vi "BlueSimpleReachTask - Front panel timer.vi"() -> ()   [LabVIEW 2010]
uses:
  Controls/Bits to Write.ctl
panel:
  in  "Use Arm Freeze Counter":bool
  out "Arm Freeze Counter":dbl
  in  "Catch probability":i32 min=0 max=100 step=1
  out "Catch Trial?":bool
  in  "Catch Trial":bool
  out "DO Task":refnum<k21>="BlueSimple_DO_All"
  out "DI Task":refnum<k21>="BlueSimple_DI"
  out "Exp correct":i32
  out "Record flag":bool
  in  "Recenter motor":bool
  in  "Override bumps":bool
  in  "Start bump timer?":bool
  in  "Trial type":u16(ring) items=["Allflash/sensory", "Precue/memory"]
  in  "DBS On?":bool
  in  "Home+target OK?":bool
  out "Exp reset":bool
  out "target set #":i32
  in  "duration (s)":dbl=0.18 format="%.4f"
  in  "Inter-pulse delay":cluster{"Fix":dbl, "Rnd":dbl}={"Fix"=0.0, "Rnd"=1.5} {"Rnd" format="%.4f"; "Fix" format="%_4g"}
  in  "Autofeed?":bool
  out "Just initialized\nhold loop?":bool
  in  "Home reward?":bool
  in  "Home reward":cluster{"Fix":dbl, "Rnd":dbl} {"Rnd" format="%.4f"; "Fix" format="%_4g"}
  in  "Override 4":bool caption="Override 1"
  in  "Override 3":bool caption="Override 1"
  in  "Override 2":bool=TRUE caption="Override 1"
  in  "Override 1":bool=TRUE
  in  "LED lines":T1={"LED1"=1, "LED2"=2, "LED3"=3, "LED4"=4}
  in  "LED1":i16=5
  in  "LED2":i16=6
  in  "LED3":i16=7
  in  "LED4":i16=8
  in  "Bump Parameters":T2={"Distance (deg)"=2.0, "Travel time (ms)"=500.0} {"Travel time (ms)" min=0.1 max=10000.0; "Distance (deg)" min=0.1}
  in  "Bump delay":cluster{"Fix":dbl, "Rnd":dbl}={"Fix"=2.0, "Rnd"=8.0} {"Rnd" format="%.4f"; "Fix" format="%_4g"}
  in  "Sine parameters":T3={"Frequency"=1.0, "Degrees\npk-pk"=8.0, "Cycles"=10000} {"Degrees\npk-pk" min=0.1 max=120.0; "Frequency" min=0.001 format="%#_4g"}
  in  "Home":bool
  in  "Bumps":bool
  in  "Sines?":bool
  out "target set size":i32
  out "# target sets":u16
  in  "# Cycles":i16=20
  out "Instruct duration":dbl format="%.4f"
  out "Pre-I hold":dbl format="%.4f"
  out "Touching target\nlast time?":bool
  in  "Rand/Seq?":bool=TRUE
  in  "Target set":i16[](array[ring]) items=["1", "2", "3", "4"]
  in  "Block":T4(array[cluster])=array[6501 elements]
  in  "Settings In":T5={"Pre-I hold"={"Fixed (s)"=0.5, "Random (s)"=0.5}, "LED I duration"={"Fixed (s)"=0.5, "Random (s)"=0.0}, "All Flash?"=FALSE, "Pre-cue brightness"=0, "Post-I hold"={"Fixed (s)"=0.7, "Random (s)"=0.3}, "Post-I \nbounce-off"={"Fixed (s)"=0.3, "Random (s)"=0.0}, "Capture timeout"={"Fixed (s)"=1.5, "Random (s)"=0.0}, "Tone duration"={"Fixed (s)"=0.5, "Random (s)"=0.0}, "LED C duration"={"Fixed (s)"=0.5, "Random (s)"=0.0}, "Cue brightness"=0, "Hold duration"={"Fixed (s)"=0.3, "Random (s)"=0.0}, "Allowed\nbounce-off"={"Fixed (s)"=0.2, "Random (s)"=0.0}, "Post-capture brightness"=0, "Reward duration"={"Fixed (s)"=0.7, "Random (s)"=0.0}, "Intertrial interval"={"Fixed (s)"=0.5, "Random (s)"=0.0}, "Persistent Mode?"=FALSE, "Error bong?"=TRUE, "Critter"=0, "Blocks"=[], "Target set"=[], "Rand/Seq?"=TRUE, "Trial type"=0, "Sines?"=FALSE, "Bumps"=FALSE, "Sine parameters"={"Frequency"=0.25, "Degrees\npk-pk"=6.0, "Cycles"=10000}, "Bump timing"={"Fix"=2.0, "Rnd"=8.0}, "Bump Parameters"={"Distance (deg)"=2.0, "Travel time (ms)"=500.0}, "DBS On?"=FALSE, "Home reward?"=FALSE, "Home+target OK?"=FALSE} {"Bump Parameters"."Travel time (ms)" min=0.1 max=10000.0; "Bump Parameters"."Distance (deg)" min=0.1; "Bump timing"."Rnd" format="%.4f"; "Bump timing"."Fix" format="%_4g"; "Sine parameters"."Degrees\npk-pk" min=0.1 max=120.0; "Sine parameters"."Frequency" min=0.001 format="%#_4g"; "Trial type" items=["Allflash/sensory", "Precue/memory"]; "Target set" items=["1", "2", "3", "4"]; "Critter" items=["Mojo", "Smokey"]; "Post-I \nbounce-off"."Random (s)" format="%.4f"; "Post-I \nbounce-off"."Fixed (s)" format="%_4g"; "Allowed\nbounce-off"."Random (s)" format="%.4f"; "Allowed\nbounce-off"."Fixed (s)" format="%_4g"; "LED C duration"."Random (s)" format="%.4f"; "LED C duration"."Fixed (s)" format="%.4f"; "Capture timeout"."Random (s)" format="%.4f"; "Capture timeout"."Fixed (s)" format="%.4f"; "Post-I hold"."Random (s)" format="%.4f"; "Post-I hold"."Fixed (s)" format="%.4f"; "Hold duration"."Random (s)" format="%.4f"; "Hold duration"."Fixed (s)" format="%_4g"; "Intertrial interval"."Random (s)" format="%.4f"; "Intertrial interval"."Fixed (s)" format="%.4f"; "Reward duration"."Random (s)" format="%.4f"; "Reward duration"."Fixed (s)" format="%.4f"; "LED I duration"."Random (s)" format="%.4f"; "LED I duration"."Fixed (s)" format="%.4f"; "Tone duration"."Random (s)" format="%.4f"; "Tone duration"."Fixed (s)" format="%.4f"; "Pre-I hold"."Random (s)" format="%.4f"; "Pre-I hold"."Fixed (s)" format="%_4g"}
  in  "pause":bool
  out "Assign settings":bool
  out "current path":path
  out "next trial path":path
  in  "Critter":u16(ring) items=["Mojo", "Smokey", "Blue", "Odo", "Monk 5", "Monk 6", "Monk 7", "Monk 8", "Monk 9", "Monk 10"]
  out "Total incorrect":i32
  in  "Write Settings":bool
  in  "Read Settings":bool
  in  "All Flash?":bool
  in  "Post-capture brightness":i16 caption="Brightness"
  in  "Cue brightness":i16=6 caption="Brightness"
  in  "Pre-cue brightness":i16 caption="Brightness"
  out "Total correct":i32
  out "Total %":dbl
  out "Total trials":i32
  in  "Error\nbong?":bool=TRUE
  out "TS Home":bool
  out "TS 4":bool
  out "TS 3":bool
  out "TS 2":bool
  out "TS 1":bool
  out "Waveform Chart":T6(graph)
  out "Block trials":i32
  out "Block %":dbl
  in  "Reset\ncounters":bool
  in  "Post-I \nbounce-off":cluster{"Fix":dbl, "Rnd":dbl}={"Fix"=0.3, "Rnd"=0.0} caption="Allowed\nbounce-off" {"Rnd" format="%.4f"; "Fix" format="%_4g"}
  out "Exp trials":i32
  out "Exp %":dbl
  in  "Touch lines":T7={"Home touch"=0, "Touch 1"=1, "Touch 2"=2, "Touch 3"=3, "Touch 4"=4}
  out "Current stage":T8(ring)
  in  "Allowed\nbounce-off":cluster{"Fix":dbl, "Rnd":dbl}={"Fix"=0.2, "Rnd"=0.0} {"Rnd" format="%.4f"; "Fix" format="%_4g"}
  in  "LED C duration":cluster{"Fix":dbl, "Rnd":dbl}={"Fix"=0.5, "Rnd"=0.0} caption="LED duration" {"Rnd" format="%.4f"; "Fix" format="%.4f"}
  in  "Capture timeout":cluster{"Fix":dbl, "Rnd":dbl}={"Fix"=1.5, "Rnd"=0.0} caption="Response time" {"Rnd" format="%.4f"; "Fix" format="%.4f"}
  in  "Post-I hold":cluster{"Fix":dbl, "Rnd":dbl}={"Fix"=0.5, "Rnd"=0.5} {"Rnd" format="%.4f"; "Fix" format="%.4f"}
  out "Last trial successful?":bool
  in  "Persistent\n Mode?":bool
  in  "Touch 4":i16=4
  in  "Touch 3":i16=3
  in  "Touch 2":i16=2
  in  "Touch 1":i16=1
  in  "Home touch":i16
  in  "Hold duration":cluster{"Fix":dbl, "Rnd":dbl}={"Fix"=0.3, "Rnd"=0.0} {"Rnd" format="%.4f"; "Fix" format="%_4g"}
  out "Target":i16
  in  "stop":bool
  in  "device":i16=1
  in  "line direction map":i32=2147483616 format="%.0b"
  out "DIGIO task ID":u32 format="%.0x"
  out "error out":errorcluster
  in  "Intertrial interval":cluster{"Fix":dbl, "Rnd":dbl}={"Fix"=0.5, "Rnd"=0.0} {"Rnd" format="%.4f"; "Fix" format="%.4f"}
  in  "Reward duration":cluster{"Fix":dbl, "Rnd":dbl}={"Fix"=0.7, "Rnd"=0.0} {"Rnd" format="%.4f"; "Fix" format="%.4f"}
  in  "LED I duration":cluster{"Fix":dbl, "Rnd":dbl}={"Fix"=0.5, "Rnd"=0.0} caption="LED duration" {"Rnd" format="%.4f"; "Fix" format="%.4f"}
  in  "Tone duration":cluster{"Fix":dbl, "Rnd":dbl}={"Fix"=0.5, "Rnd"=0.0} {"Rnd" format="%.4f"; "Fix" format="%.4f"}
  in  "Pre-I hold":cluster{"Fix":dbl, "Rnd":dbl}={"Fix"=0.5, "Rnd"=0.5} {"Rnd" format="%.4f"; "Fix" format="%_4g"}
  # "Auto-feed"
  # "DBS"
  # "Pre-\ninstruction\nhold"
  # "Post-\ninstruction\nhold"
  # "Instruction"
  # "Target capture"
  # "Target hold"
  # "Reward"
  # "Intertrial"
  # "Motor"
  # "Override"
  # "+"
  # "+"
  # "+"
  # "Pre-\ninstruction\nhold"
  # "Instruction"
  # "Post-\ninstruction\nhold"
  # "Target capture"
  # "Target hold"
  # "Reward"
  # "Intertrial"
  # "+"
  # "+"
  # "+"
  # "+"
  # "+"
  # "+"
  # "+"
  # "+"
  # "+"
  # "+"
  # "+"
  # "+"
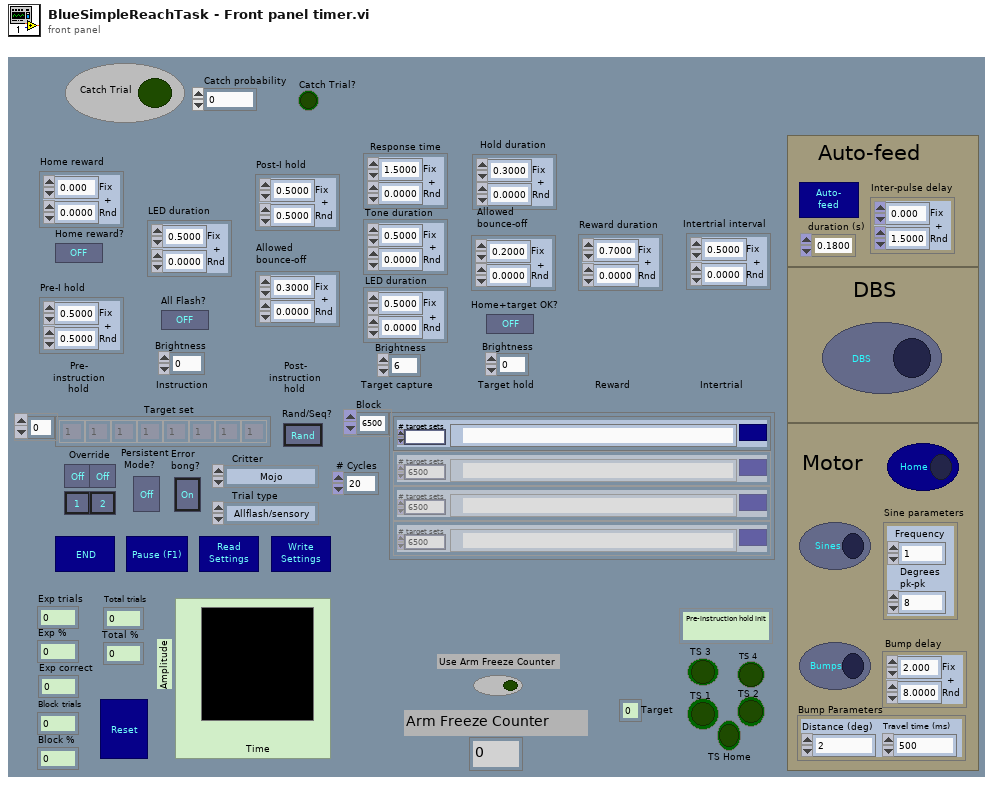
[diagram p1: front panel]
types:
  T1 = cluster{"LED1":i16, "LED2":i16, "LED3":i16, "LED4":i16}
  T2 = cluster{"Distance (deg)":dbl, "Travel time (ms)":dbl}
  T3 = cluster{"Frequency":dbl, "Degrees\npk-pk":dbl, "Cycles":i16}
  T4 = cluster{"Settings file":path, "# target sets":u16}[]
  T5 = cluster{"Pre-I hold":cluster{"Fixed (s)":dbl, "Random (s)":dbl}, "LED I duration":cluster{"Fixed (s)":dbl, "Random (s)":dbl}, "All Flash?":bool, "Pre-cue brightness":i16, "Post-I hold":cluster{"Fixed (s)":dbl, "Random (s)":dbl}, "Post-I \nbounce-off":cluster{"Fixed (s)":dbl, "Random (s)":dbl}, "Capture timeout":cluster{"Fixed (s)":dbl, "Random (s)":dbl}, "Tone duration":cluster{"Fixed (s)":dbl, "Random (s)":dbl}, "LED C duration":cluster{"Fixed (s)":dbl, "Random (s)":dbl}, "Cue brightness":i16, "Hold duration":cluster{"Fixed (s)":dbl, "Random (s)":dbl}, "Allowed\nbounce-off":cluster{"Fixed (s)":dbl, "Random (s)":dbl}, "Post-capture brightness":i16, "Reward duration":cluster{"Fixed (s)":dbl, "Random (s)":dbl}, "Intertrial interval":cluster{"Fixed (s)":dbl, "Random (s)":dbl}, "Persistent Mode?":bool, "Error bong?":bool, "Critter":u16, "Blocks":cluster{"Settings file":path, "# target sets":dbl}[], "Target set":i16[], "Rand/Seq?":bool, "Trial type":u16, "Sines?":bool, "Bumps":bool, "Sine parameters":cluster{"Frequency":dbl, "Degrees\npk-pk":dbl, "Cycles":i16}, "Bump timing":cluster{"Fix":dbl, "Rnd":dbl}, "Bump Parameters":cluster{"Distance (deg)":dbl, "Travel time (ms)":dbl}, "DBS On?":bool, "Home reward?":bool, "Home+target OK?":bool}
  T6 = cluster{"Segment Percentage":dbl, "Total % correct":dbl}
  T7 = cluster{"Home touch":i16, "Touch 1":i16, "Touch 2":i16, "Touch 3":i16, "Touch 4":i16}
  T8 = enum16{"Pre-instruction hold init", "Pre-instruction hold", "Instruction init", "Instruction", "Post-instruction hold init", "Post-instruction hold", "Target capture init", "Target capture", "Target hold init", "Target hold", "Reward stage", "Intertrial"}
  T9 = typedef "Bits to Write.ctl" = enum16{"LED 1 on", "LED 1 off", "LED 2 on", "LED 2 off", "LED 3 on", "LED 3 off", "LED 4 on", "LED 4 off", "All LEDs on", "All LEDs off", "In trial on", "In trial off", "Buzzer on", "Buzzer off", "Reward on", "Reward off", "Target number", "Trial type preQ on", "Trial type preQ off", "Error on", "Error off", "Trial number", "DBS on", "DBS off", "Sine on", "Sine off", "All Bits On", "All Bits Off", "Init", "Specify mask/pattern"}
  T10 = enum16{"Reset", "Increment", "Reset for exp", "Initialize"}
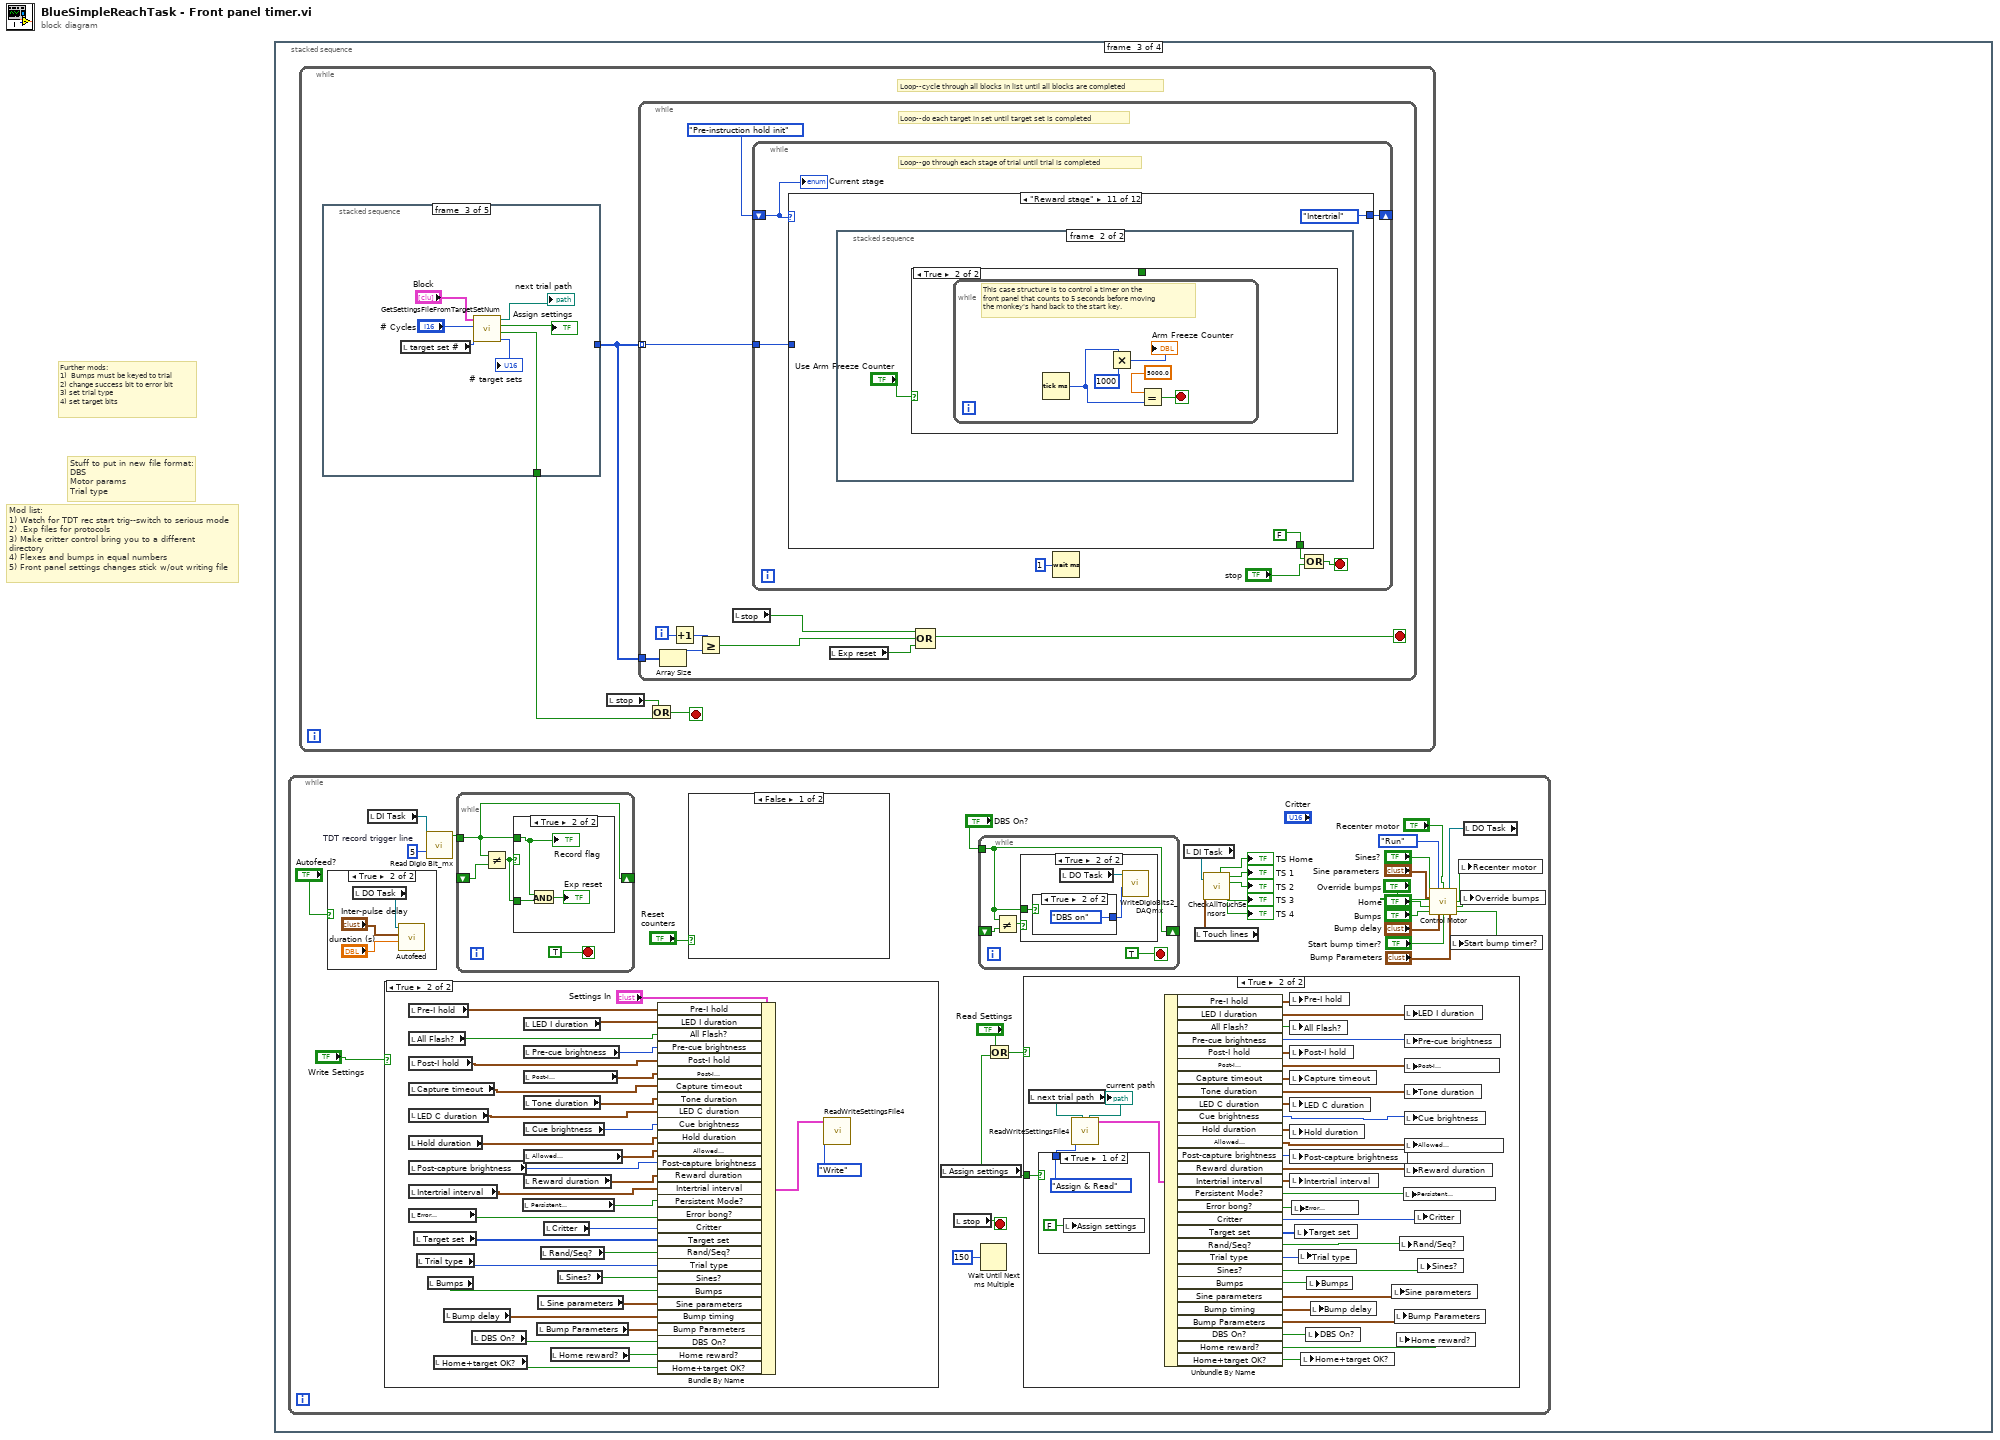
[diagram p0: block diagram]
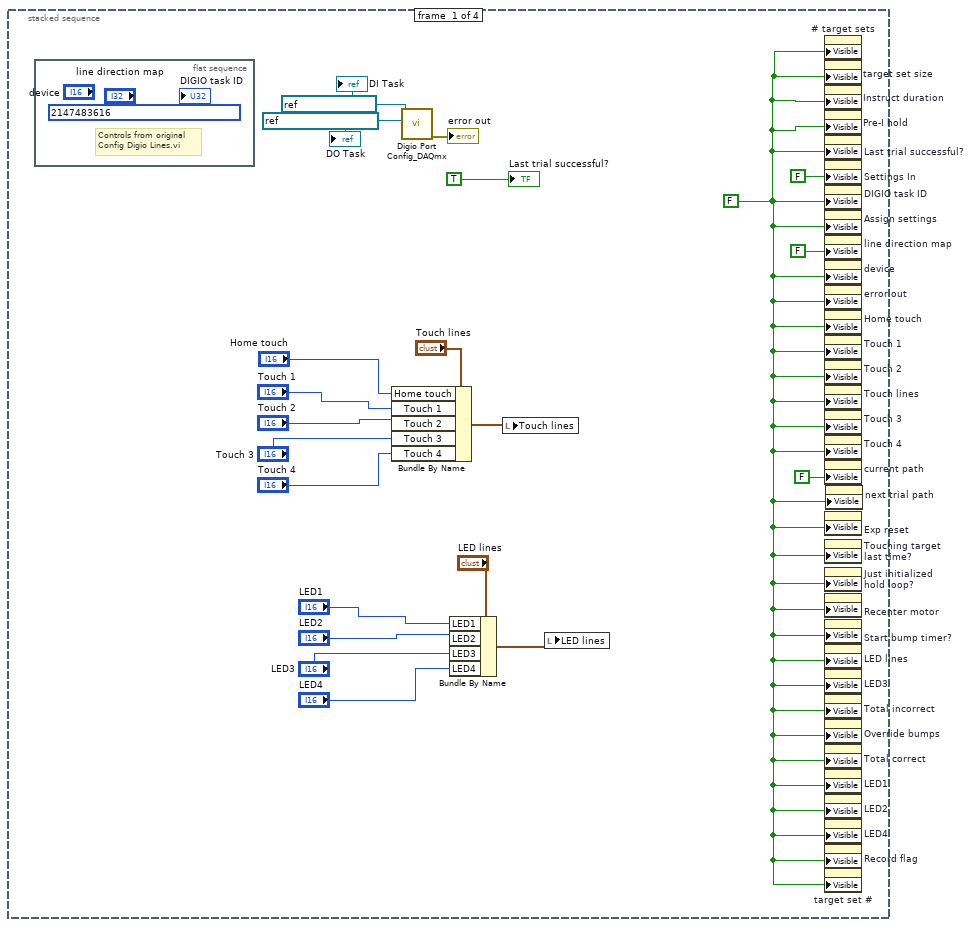
[diagram p2: hidden frame]
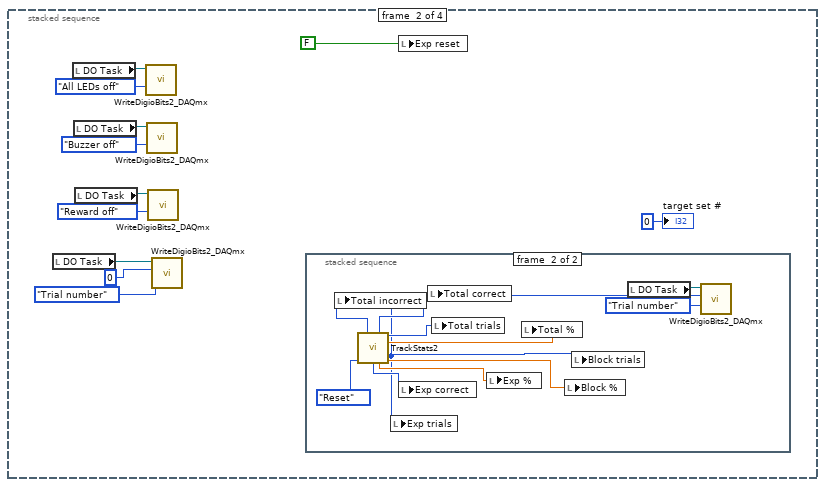
[diagram p3: hidden frame]
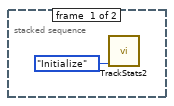
[diagram p4: hidden frame]
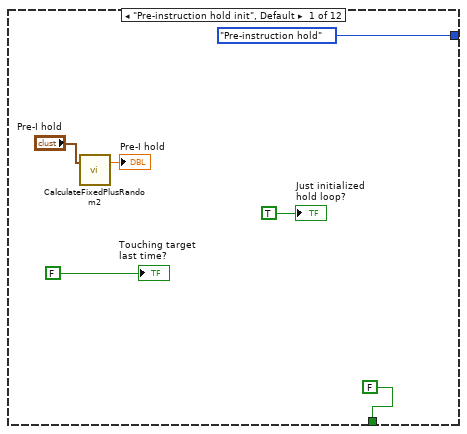
[diagram p5: hidden frame]
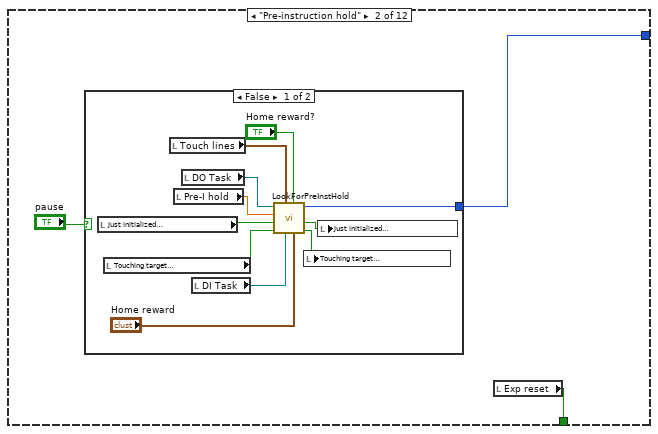
[diagram p6: hidden frame]
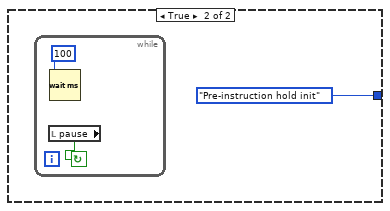
[diagram p7: hidden frame]
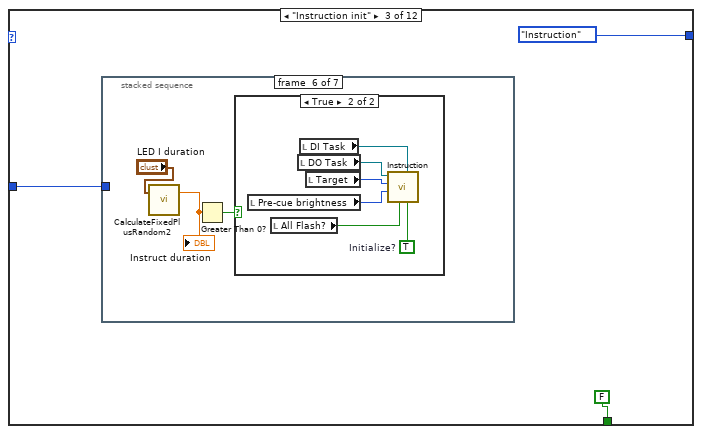
[diagram p8: hidden frame]
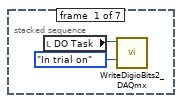
[diagram p9: hidden frame]
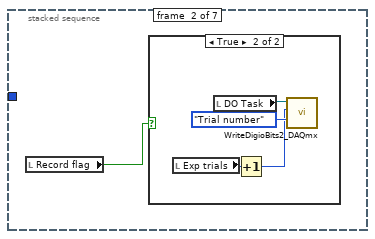
[diagram p10: hidden frame]
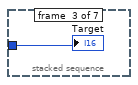
[diagram p12: hidden frame]
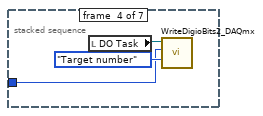
[diagram p13: hidden frame]
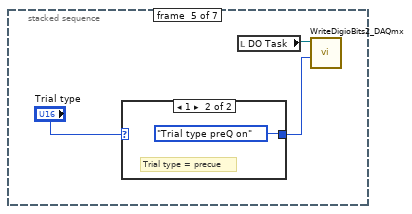
[diagram p14: hidden frame]
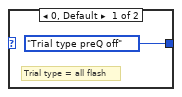
[diagram p15: hidden frame]
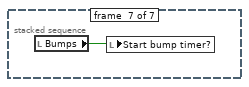
[diagram p17: hidden frame]
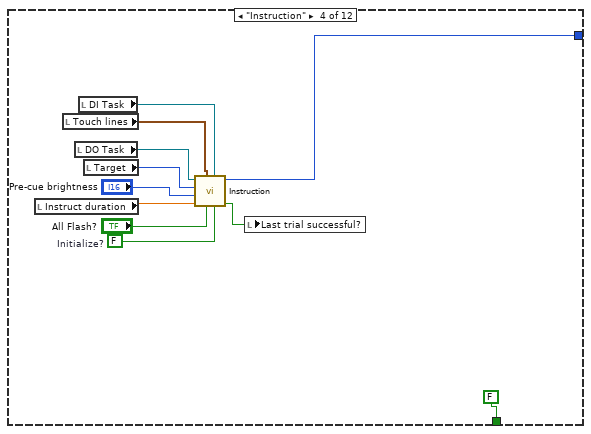
[diagram p18: hidden frame]
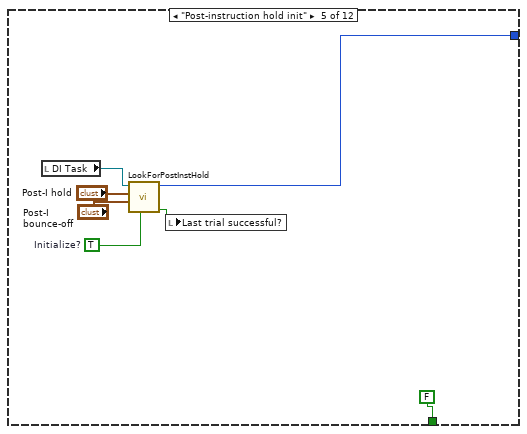
[diagram p19: hidden frame]
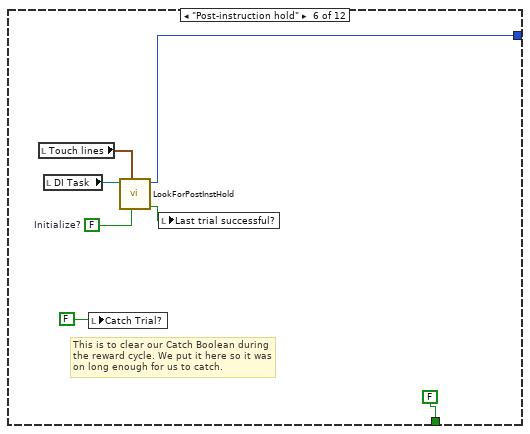
[diagram p20: hidden frame]
diagram:
  # "Stuff to put in new file format:\nDBS\nMotor params\nTrial type"
  # "Further mods:\n1)  Bumps must be keyed to trial\n2) change success bit to error bit\n3) set trial type\n4) set target bits"
  # "Mod list:\n1) Watch for TDT rec start trig--switch to serious mode\n2) .Exp files for protocols\n3) Make critter control bring you to a different directory\n4) Flexes and bumps in equal numbers\n5) Front panel settings changes stick w/out writing file"
  n1 = stacked-sequence {
    frame #0 {
      w2 = refnum<k21> "BlueSimple_DO_All" ("DO Task")
      w3 = refnum<k21> "BlueSimple_DI" ("DI Task")
      w4 = FALSE ("Persistent Mode?")
      n2 = flat-sequence {
        frame #0 {
          (unwired) 2147483616 ("line direction map")
          # "Controls from original\nConfig Digio Lines.vi"
        }
      }
      n3 = Bundle By Name(cluster="Touch lines", "Home touch"="Home touch", "Touch 1"="Touch 1", "Touch 2"="Touch 2", "Touch 3"="Touch 3", "Touch 4"="Touch 4") -> (w20:T7)
      n4 = call "Digio Port Config_DAQmx.vi"("DO Task"=w2, "DI Task"=w3) -> ("error out"=→"error out":errorcluster)  [unwired: 7 in]
      n5 = Bundle By Name(cluster="LED lines", "LED1"="LED1", "LED2"="LED2", "LED3"="LED3", "LED4"="LED4") -> (w8:T1)
      n6 = local write "Touch lines"(w20) -> ()
      n7 = local write "LED lines"(w8) -> ()
      n8 = property on="# target sets" class="DigNum (strict)"("Visible"=w4) -> ()  [unwired: 2 in, 2 out]
      n9 = property on="target set size" class="DigNum (strict)"("Visible"=w4) -> ()  [unwired: 2 in, 2 out]
      n10 = property on="Instruct duration" class="DigNum (strict)"("Visible"=w4) -> ()  [unwired: 2 in, 2 out]
      n11 = property on="Pre-I hold" class="DigNum (strict)"("Visible"=w4) -> ()  [unwired: 2 in, 2 out]
      n12 = property on="Last trial successful?" class="Bool (strict)"("Visible"=w4) -> ()  [unwired: 2 in, 2 out]
      n13 = property on="Settings In" class="Clust (strict)"("Visible"=FALSE) -> ()  [unwired: 2 in, 2 out]
      n14 = property on="DIGIO task ID" class="DigNum (strict)"("Visible"=w4) -> ()  [unwired: 2 in, 2 out]
      n15 = property on="Assign settings" class="Bool (strict)"("Visible"=w4) -> ()  [unwired: 2 in, 2 out]
      n16 = property on="line direction map" class="DigNum (strict)"("Visible"=FALSE) -> ()  [unwired: 2 in, 2 out]
      n17 = property on="device" class="DigNum (strict)"("Visible"=w4) -> ()  [unwired: 2 in, 2 out]
      n18 = property on="error out" class="Clust (strict)"("Visible"=w4) -> ()  [unwired: 2 in, 2 out]
      n19 = property on="Home touch" class="DigNum (strict)"("Visible"=w4) -> ()  [unwired: 2 in, 2 out]
      n20 = property on="Touch 1" class="DigNum (strict)"("Visible"=w4) -> ()  [unwired: 2 in, 2 out]
      n21 = property on="Touch 2" class="DigNum (strict)"("Visible"=w4) -> ()  [unwired: 2 in, 2 out]
      n22 = property on="Touch lines" class="Clust (strict)"("Visible"=w4) -> ()  [unwired: 2 in, 2 out]
      n23 = property on="Touch 3" class="DigNum (strict)"("Visible"=w4) -> ()  [unwired: 2 in, 2 out]
      n24 = property on="Touch 4" class="DigNum (strict)"("Visible"=w4) -> ()  [unwired: 2 in, 2 out]
      n25 = property on="current path" class="Path"("Visible"=FALSE) -> ()  [unwired: 2 in, 2 out]
      n26 = property on="Exp reset" class="Bool (strict)"("Visible"=w4) -> ()  [unwired: 2 in, 2 out]
      n27 = property on="Touching target\nlast time?" class="Bool (strict)"("Visible"=w4) -> ()  [unwired: 2 in, 2 out]
      n28 = property on="Just initialized\nhold loop?" class="Bool (strict)"("Visible"=w4) -> ()  [unwired: 2 in, 2 out]
      n29 = property on="Recenter motor" class="Bool (strict)"("Visible"=w4) -> ()  [unwired: 2 in, 2 out]
      n30 = property on="Start bump timer?" class="Bool (strict)"("Visible"=w4) -> ()  [unwired: 2 in, 2 out]
      n31 = property on="LED lines" class="Clust (strict)"("Visible"=w4) -> ()  [unwired: 2 in, 2 out]
      n32 = property on="LED3" class="DigNum (strict)"("Visible"=w4) -> ()  [unwired: 2 in, 2 out]
      n33 = property on="Total incorrect" class="DigNum (strict)"("Visible"=w4) -> ()  [unwired: 2 in, 2 out]
      n34 = property on="Override bumps" class="Bool (strict)"("Visible"=w4) -> ()  [unwired: 2 in, 2 out]
      n35 = property on="Total correct" class="DigNum (strict)"("Visible"=w4) -> ()  [unwired: 2 in, 2 out]
      n36 = property on="LED1" class="DigNum (strict)"("Visible"=w4) -> ()  [unwired: 2 in, 2 out]
      n37 = property on="LED2" class="DigNum (strict)"("Visible"=w4) -> ()  [unwired: 2 in, 2 out]
      n38 = property on="LED4" class="DigNum (strict)"("Visible"=w4) -> ()  [unwired: 2 in, 2 out]
      n39 = property on="Record flag" class="Bool (strict)"("Visible"=w4) -> ()  [unwired: 2 in, 2 out]
      n40 = property on="target set #" class="DigNum (strict)"("Visible"=w4) -> ()  [unwired: 2 in, 2 out]
      n41 = property on="next trial path" class="Path"("Visible"=w4) -> ()  [unwired: 2 in, 2 out]
      "Last trial successful?" <- TRUE ("Persistent Mode?")
      "DI Task" <- w3
      "DO Task" <- w2
    }
    frame #1 {
      n42 = local read "DO Task"() -> (w30:refnum<k21>)
      n43 = local read "DO Task"() -> (w23:refnum<k21>)
      n44 = local read "DO Task"() -> (w24:refnum<k21>)
      n45 = local read "DO Task"() -> (w26:refnum<k21>)
      n46 = call "WriteDigioBits2_DAQmx.vi"("Bits to write"=Bits_to_Write."All LEDs off", "DO Task"=w23) -> ()  [unwired: 9 in, 1 out]
      n47 = call "WriteDigioBits2_DAQmx.vi"("Bits to write"=Bits_to_Write."Buzzer off", "DO Task"=w24) -> ()  [unwired: 9 in, 1 out]
      n48 = call "WriteDigioBits2_DAQmx.vi"("Bits to write"=Bits_to_Write."Reward off", "DO Task"=w26) -> ()  [unwired: 9 in, 1 out]
      n49 = call "WriteDigioBits2_DAQmx.vi"("Bits to write"=Bits_to_Write."Trial number", "Number"=u32 0, "DO Task"=w30) -> ()  [unwired: 8 in, 1 out]
      n50 = stacked-sequence {
        frame #0 {
          n51 = call "TrackStats2.vi"("Command"=T10."Initialize") -> ()  [unwired: 6 in, 9 out]
        }
        frame #1 {
          n52 = call "TrackStats2.vi"("Command"=T10."Reset") -> ("Total incorrect"=w45:i32, "Total correct"=w44:i32, "# total trials"=w43:i32, "Total % correct"=w42:dbl, "Segment trials"=w38:i32, "Experiment trials"=w34:i32, "Experiment correct"=w37:i32, "Experiment %"=w40:dbl, "Segment Percentage"=w41:dbl)  [unwired: 6 in]
          n53 = local write "Total incorrect"(w45) -> ()
          n54 = local write "Exp trials"(w34) -> ()
          n55 = local write "Exp correct"(w37) -> ()
          n56 = local write "Total correct"(w44) -> ()
          n57 = local write "Total trials"(w43) -> ()
          n58 = local write "Exp %"(w40) -> ()
          n59 = local write "Total %"(w42) -> ()
          n60 = local write "Block %"(w41) -> ()
          n61 = local write "Block trials"(w38) -> ()
          n62 = local read "DO Task"() -> (w36:refnum<k21>)
          n63 = call "WriteDigioBits2_DAQmx.vi"("Bits to write"=Bits_to_Write."Trial number", "Number"=w34, "DO Task"=w36) -> ()  [unwired: 8 in, 1 out]
        }
      }
      n64 = local write "Exp reset"(FALSE ("Exp reset")) -> ()
      "target set #" <- 0 ("target set #")
    }
    frame #2 {
      n65 = while {
        stop <- w311 stop-if-true
        w281 = i16 5  # TDT record trigger line
        n66 = case shown="True" "Autofeed?" {
          frame False {
          }
          frame True {
            n67 = local read "DO Task"() -> (w321:refnum<k21>)
            n68 = call "Autofeed.vi"("duration"="duration (s)", "Auto-feed"="Inter-pulse delay", "DO Task"=w321) -> ()  [unwired: 4 in]
          }
        }
        n69 = local read "DI Task"() -> (w280:refnum<k21>)
        n70 = case shown="True" "Write Settings" {
          frame False {
          }
          frame True {
            n71 = local read "Pre-I hold"() -> (w362:cluster{"Fix":dbl, "Rnd":dbl})
            n72 = local read "All Flash?"() -> (w360:bool)
            n73 = local read "Post-I hold"() -> (w358:cluster{"Fix":dbl, "Rnd":dbl})
            n74 = local read "Capture timeout"() -> (w356:cluster{"Fix":dbl, "Rnd":dbl})
            n75 = local read "LED C duration"() -> (w354:cluster{"Fix":dbl, "Rnd":dbl})
            n76 = local read "Hold duration"() -> (w352:cluster{"Fix":dbl, "Rnd":dbl})
            n77 = local read "Post-capture brightness"() -> (w350:i16)
            n78 = local read "Intertrial interval"() -> (w348:cluster{"Fix":dbl, "Rnd":dbl})
            n79 = local read "Error\nbong?"() -> (w346:bool)
            n80 = local read "Target set"() -> (w342:i16[])
            n81 = local read "Trial type"() -> (w339:u16)
            n82 = local read "Bumps"() -> (w337:bool)
            n83 = local read "Home+target OK?"() -> (w331:bool)
            n84 = local read "Bump delay"() -> (w335:cluster{"Fix":dbl, "Rnd":dbl})
            n85 = local read "DBS On?"() -> (w333:bool)
            n86 = local read "Persistent\n Mode?"() -> (w347:bool)
            n87 = local read "LED I duration"() -> (w361:cluster{"Fix":dbl, "Rnd":dbl})
            n88 = local read "Pre-cue brightness"() -> (w359:i16)
            n89 = local read "Post-I \nbounce-off"() -> (w357:cluster{"Fix":dbl, "Rnd":dbl})
            n90 = local read "Tone duration"() -> (w355:cluster{"Fix":dbl, "Rnd":dbl})
            n91 = local read "Cue brightness"() -> (w353:i16)
            n92 = local read "Allowed\nbounce-off"() -> (w351:cluster{"Fix":dbl, "Rnd":dbl})
            n93 = local read "Reward duration"() -> (w349:cluster{"Fix":dbl, "Rnd":dbl})
            n94 = local read "Bump Parameters"() -> (w334:T2)
            n95 = local read "Sine parameters"() -> (w336:T3)
            n96 = local read "Rand/Seq?"() -> (w341:bool)
            n97 = local read "Critter"() -> (w343:u16)
            n98 = local read "Home reward?"() -> (w332:bool)
            n99 = local read "Sines?"() -> (w338:bool)
            n100 = Bundle By Name(cluster="Settings In", "Pre-I hold"=w362, "LED I duration"=w361, "All Flash?"=w360, "Pre-cue brightness"=w359, "Post-I hold"=w358, "Post-I \nbounce-off"=w357, "Capture timeout"=w356, "Tone duration"=w355, "LED C duration"=w354, "Cue brightness"=w353, "Hold duration"=w352, "Allowed\nbounce-off"=w351, "Post-capture brightness"=w350, "Reward duration"=w349, "Intertrial interval"=w348, "Persistent Mode?"=w347, "Error bong?"=w346, "Critter"=w343, "Target set"=w342, "Rand/Seq?"=w341, "Trial type"=w339, "Sines?"=w338, "Bumps"=w337, "Sine parameters"=w336, "Bump timing"=w335, "Bump Parameters"=w334, "DBS On?"=w333, "Home reward?"=w332, "Home+target OK?"=w331) -> (w340:T5)
            n101 = call "ReadWriteSettingsFile4.vi"("Read/write"=enum16{"Query & Read", "Assign & Read", "Write"}."Write", "Settings In"=w340) -> ()  [unwired: 4 in, 4 out]
          }
        }
        n102 = call "Read Digio Bit_mx.vi"("line"=w281, "DI Task"=w280) -> ("line state"=w279:bool)  [unwired: 7 in, 1 out]
        n103 = while {
          tunnel: w279 -> [w325]
          shift-right: [w325] -> _
          shift-left: _ -> [w326]
          stop <- TRUE stop-if-true
          n104 = Not Equal?(x=w325, y=w326) -> (x != y?=w324:bool)
          n105 = case shown="True" w324 {
            tunnel: w325 -> [_ w328]
            tunnel: w324 -> [_ w329]
            frame False {
            }
            frame True {
              n106 = And(x=w328, y=w329) -> (x .and. y?=→"Exp reset":bool)
              "Record flag" <- w328
            }
          }
        }
        n107 = case shown="False" "Reset\ncounters" {
          frame False {
          }
          frame True {
            n108 = call "TrackStats2.vi"("Command"=T10."Reset") -> ("Total incorrect"=w408:i32, "Total correct"=w407:i32, "# total trials"=w406:i32, "Total % correct"=w405:dbl, "Segment trials"=w404:i32, "Experiment trials"=w401:i32, "Experiment %"=w402:dbl, "Segment Percentage"=w403:dbl)  [unwired: 6 in, 1 out]
            n109 = local write "Total incorrect"(w408) -> ()
            n110 = local write "Total correct"(w407) -> ()
            n111 = local write "Exp trials"(w401) -> ()
            n112 = local write "Exp %"(w402) -> ()
            n113 = local write "Block %"(w403) -> ()
            n114 = local write "Block trials"(w404) -> ()
            n115 = local write "Total trials"(w406) -> ()
            n116 = local write "Total %"(w405) -> ()
          }
        }
        n117 = local read "Assign settings"() -> (w299:bool)
        n118 = local read "stop"() -> (w311:bool)
        n119 = while {
          shift-right: [w313] -> _
          shift-left: _ -> [w314]
          tunnel: "DBS On?" -> [w313]
          stop <- TRUE stop-if-true
          n120 = Not Equal?(x=w313, y=w314) -> (x != y?=w312:bool)
          n121 = case shown="True" w312 {
            tunnel: w313 -> [_ w318]
            frame False {
            }
            frame True {
              n122 = case shown="True" w318 {
                tunnel: [Bits_to_Write."DBS off" ("Bits to write") Bits_to_Write."DBS on" ("Bits to write")] -> w316
                frame False {
                }
                frame True {
                }
              }
              n123 = local read "DO Task"() -> (w317:refnum<k21>)
              n124 = call "WriteDigioBits2_DAQmx.vi"("Bits to write"=w316, "DO Task"=w317) -> ()  [unwired: 9 in, 1 out]
            }
          }
        }
        n125 = Wait Until Next ms Multiple(millisecond multiple=u32 150) -> ()  [unwired: 1 out]
        n126 = Or(x="Read Settings", y=w299) -> (x .or. y?=w300:bool)
        n127 = case shown="True" w300 {
          tunnel: w299 -> [_ w375]
          frame False {
          }
          frame True {
            n128 = local read "next trial path"() -> (w376:path)
            n129 = case shown="True" w375 {
              tunnel: [enum16{"Query & Read", "Assign & Read", "Write"}."Assign & Read" ("Read/write") enum16{"Query & Read", "Assign & Read", "Write"}."Query & Read" ("Read/write")] -> w378
              frame True {
                n130 = local write "Assign settings"(FALSE ("Assign settings")) -> ()
              }
              frame False {
              }
            }
            n131 = call "ReadWriteSettingsFile4.vi"("file path"=w376, "Read/write"=w378) -> ("Settings Out"=w396:T5, "current path"=→"current path":path)  [unwired: 4 in, 2 out]
            n132 = Unbundle By Name(w396) -> ("Pre-I hold"=w395:cluster{"Fixed (s)":dbl, "Random (s)":dbl}, "LED I duration"=w394:cluster{"Fixed (s)":dbl, "Random (s)":dbl}, "All Flash?"=w393:bool, "Pre-cue brightness"=w392:i16, "Post-I hold"=w391:cluster{"Fixed (s)":dbl, "Random (s)":dbl}, "Post-I \nbounce-off"=w390:cluster{"Fixed (s)":dbl, "Random (s)":dbl}, "Capture timeout"=w389:cluster{"Fixed (s)":dbl, "Random (s)":dbl}, "Tone duration"=w388:cluster{"Fixed (s)":dbl, "Random (s)":dbl}, "LED C duration"=w387:cluster{"Fixed (s)":dbl, "Random (s)":dbl}, "Cue brightness"=w386:i16, "Hold duration"=w385:cluster{"Fixed (s)":dbl, "Random (s)":dbl}, "Allowed\nbounce-off"=w384:cluster{"Fixed (s)":dbl, "Random (s)":dbl}, "Post-capture brightness"=w383:i16, "Reward duration"=w382:cluster{"Fixed (s)":dbl, "Random (s)":dbl}, "Intertrial interval"=w381:cluster{"Fixed (s)":dbl, "Random (s)":dbl}, "Persistent Mode?"=w380:bool, "Error bong?"=w379:bool, "Critter"=w374:u16, "Target set"=w373:i16[], "Rand/Seq?"=w372:bool, "Trial type"=w371:u16, "Sines?"=w370:bool, "Bumps"=w369:bool, "Sine parameters"=w368:T3, "Bump timing"=w367:cluster{"Fix":dbl, "Rnd":dbl}, "Bump Parameters"=w366:T2, "DBS On?"=w365:bool, "Home reward?"=w364:bool, "Home+target OK?"=w363:bool)
            n133 = local write "Pre-I hold"(w395) -> ()
            n134 = local write "All Flash?"(w393) -> ()
            n135 = local write "Post-I hold"(w391) -> ()
            n136 = local write "Capture timeout"(w389) -> ()
            n137 = local write "LED C duration"(w387) -> ()
            n138 = local write "Hold duration"(w385) -> ()
            n139 = local write "Post-capture brightness"(w383) -> ()
            n140 = local write "Intertrial interval"(w381) -> ()
            n141 = local write "Error\nbong?"(w379) -> ()
            n142 = local write "Target set"(w373) -> ()
            n143 = local write "Trial type"(w371) -> ()
            n144 = local write "Home+target OK?"(w363) -> ()
            n145 = local write "DBS On?"(w365) -> ()
            n146 = local write "Bumps"(w369) -> ()
            n147 = local write "Bump delay"(w367) -> ()
            n148 = local write "Sine parameters"(w368) -> ()
            n149 = local write "Bump Parameters"(w366) -> ()
            n150 = local write "Home reward?"(w364) -> ()
            n151 = local write "Rand/Seq?"(w372) -> ()
            n152 = local write "Persistent\n Mode?"(w380) -> ()
            n153 = local write "LED I duration"(w394) -> ()
            n154 = local write "Pre-cue brightness"(w392) -> ()
            n155 = local write "Post-I \nbounce-off"(w390) -> ()
            n156 = local write "Tone duration"(w388) -> ()
            n157 = local write "Cue brightness"(w386) -> ()
            n158 = local write "Allowed\nbounce-off"(w384) -> ()
            n159 = local write "Reward duration"(w382) -> ()
            n160 = local write "Critter"(w374) -> ()
            n161 = local write "Sines?"(w370) -> ()
          }
        }
        n162 = local read "DI Task"() -> (w309:refnum<k21>)
        n163 = local read "Touch lines"() -> (w308:T7)
        n164 = call "CheckAllTouchSensors.vi"("Touch sensor lines"=w308, "DI Task"=w309) -> ("TS 4"=→"TS 4":bool, "TS 3"=→"TS 3":bool, "TS 2"=→"TS 2":bool, "TS 1"=→"TS 1":bool, "Home?"=→"TS Home":bool)
        n165 = local read "DO Task"() -> (w282:refnum<k21>)
        n166 = call "Control Motor.vi"("Sines?"="Sines?", "Command"=enum16{"Initialize", "Home", "Run", "Disable"}."Run", "Re-center\nmotor"="Recenter motor", "DO Task"=w282, "Sine parameters"="Sine parameters", "Override bumps"="Override bumps", "Home"="Home", "Bumps"="Bumps", "Bump timing"="Bump delay", "Start bump timer?"="Start bump timer?", "Bump Parameters"="Bump Parameters") -> ("Reset\nrecenter"=w284:bool, "Reset override bumps"=w286:bool, "Reset start button"=w288:bool)  [unwired: 2 in]
        n167 = local write "Start bump timer?"(w288) -> ()
        n168 = local write "Recenter motor"(w284) -> ()
        n169 = local write "Override bumps"(w286) -> ()
      }
      n170 = while {
        stop <- w46 stop-if-true
        # "Loop--cycle through all blocks in list until all blocks are completed"
        n171 = stacked-sequence {
          tunnel: [_ _ _ _ w266] -> w49
          tunnel: [_ _ w258 _ _] -> w47
          frame #0 {
            n172 = local read "Exp reset"() -> (w241:bool)
            n173 = case shown="True" w241 {
              frame False {
              }
              frame True {
                n174 = stacked-sequence {
                  frame #0 {
                    n175 = call <vilib>:"Beep.vi"() -> ()  [unwired: 12 in]
                    n176 = Wait (ms)(milliseconds to wait=u32 5) -> ()  [unwired: 1 out]
                  }
                  frame #1 {
                    n177 = local write "Exp reset"(FALSE ("Exp reset")) -> ()
                  }
                  frame #2 {
                    n178 = local write "target set #"(0 ("target set #")) -> ()
                  }
                  frame #3 {
                    n179 = call "TrackStats2.vi"("Command"=T10."Reset for exp") -> ("Total incorrect"=w254:i32, "Total correct"=w253:i32, "# total trials"=w252:i32, "Total % correct"=w251:dbl, "Segment trials"=w250:i32, "Experiment trials"=w247:i32, "Experiment correct"=w245:i32, "Experiment %"=w248:dbl, "Segment Percentage"=w249:dbl)  [unwired: 6 in]
                    n180 = local write "Exp trials"(w247) -> ()
                    n181 = local write "Total incorrect"(w254) -> ()
                    n182 = local write "Total correct"(w253) -> ()
                    n183 = local write "Exp %"(w248) -> ()
                    n184 = local write "Exp correct"(w245) -> ()
                    n185 = local write "Block %"(w249) -> ()
                    n186 = local write "Block trials"(w250) -> ()
                    n187 = local write "Total trials"(w252) -> ()
                    n188 = local write "Total %"(w251) -> ()
                  }
                }
              }
            }
          }
          frame #1 {
            n189 = local read "target set #"() -> (w255:i32)
            n190 = Increment(x=w255) -> (x+1=w256:i32)
            n191 = local write "target set #"(w256) -> ()
          }
          frame #2 {
            n192 = local read "target set #"() -> (w263:i32)
            n193 = call "GetSettingsFileFromTargetSetNum.vi"("target set #"=w263, "# Cycles"="# Cycles", "Block"="Block") -> ("# target sets"=→"# target sets":u16, "Completed list?"=w258:bool, "apply new settings?"=→"Assign settings":bool, "Settings file"=→"next trial path":path)  [unwired: 1 in]
          }
          frame #3 {
            n194 = local read "Assign settings"() -> (w264:bool)
            n195 = case shown="True" w264 {
              frame False {
              }
              frame True {
                # "500ms delay to allow \nsettings loop below to\ninstantiate new settings"
                n196 = Wait (ms)(milliseconds to wait=u32 500) -> ()  [unwired: 1 out]
              }
            }
          }
          frame #4 {
            n197 = call "TargetOverride.vi"("Override 1"="Override 1", "Override 2"="Override 2", "Override 3"="Override 3", "Override 4"="Override 4", "Target set"="Target set") -> ("Target set out"=w272:i16[])  [unwired: 1 in]
            n198 = case shown="True" "Rand/Seq?" {
              tunnel: w272 -> [w276 w278]
              tunnel: [w276 w277] -> w267
              frame False {
              }
              frame True {
                n199 = call "RandomizeTargetSet.vi"("Target set"=w278) -> ("Target set rand order"=w277:i16[])
              }
            }
            n200 = Increment(x=w267) -> (x+1=w266:i16[])
            n201 = Array Size(array=w266) -> (size(s)=→"target set size":i32)
          }
        }
        n202 = local read "stop"() -> (w48:bool)
        n203 = while {
          tunnel: w49 -> [w58] mode=indexing
          tunnel: w49 -> [w57]
          i -> [w56]
          stop <- w50 stop-if-true
          # "Loop--do each target in set until target set is completed"
          n204 = Array Size(array=w57) -> (size(s)=w55:i32)
          n205 = Increment(x=w56) -> (x+1=w54:i32)
          n206 = Greater Or Equal?(x=w54, y=w55) -> (x >= y?=w52:bool)
          n207 = local read "stop"() -> (w53:bool)
          n208 = while {
            shift-right: [w66] -> _
            shift-left: T8."Pre-instruction hold init" ("Current stage") -> [w65]
            tunnel: w58 -> [w64]
            stop <- w61 stop-if-true
            # "Loop--go through each stage of trial until trial is completed"
            n209 = case shown="\"Reward stage\"" w65 {
              tunnel: [T8."Pre-instruction hold" ("Current stage") w75 T8."Instruction" ("Current stage") w123 w131 w143 T8."Target capture" ("Current stage") w163 T8."Target hold" ("Current stage") w181 T8."Intertrial" ("Current stage") T8."Pre-instruction hold init" ("Current stage")] -> w66
              tunnel: [FALSE ("Just initialized\nhold loop?") w73 FALSE ("End of trial") FALSE ("End of trial") FALSE ("End of trial") FALSE ("End of trial") FALSE ("End of trial") FALSE ("End of trial") FALSE ("End of trial") FALSE ("End of trial") FALSE ("End of trial") w225] -> w63
              tunnel: w64 -> [_ _ w90 _ _ _ _ _ _ _ _ _]
              frame "Pre-instruction hold init", Default {
                n210 = call "CalculateFixedPlusRandom2.vi"("Component times"="Pre-I hold") -> ("Composite time"=→"Pre-I hold":dbl)  [unwired: 1 in, 1 out]
                "Touching target\nlast time?" <- FALSE ("Touching target\nlast time?")
                "Just initialized\nhold loop?" <- TRUE ("Just initialized\nhold loop?")
              }
              frame "Pre-instruction hold" {
                n211 = case shown="False" "pause" {
                  tunnel: [w86 T8."Pre-instruction hold init" ("Current stage")] -> w75
                  frame False {
                    n212 = local read "Just initialized\nhold loop?"() -> (w81:bool)
                    n213 = local read "Touching target\nlast time?"() -> (w83:bool)
                    n214 = local read "Touch lines"() -> (w84:T7)
                    n215 = local read "Pre-I hold"() -> (w85:dbl)
                    n216 = local read "DO Task"() -> (w77:refnum<k21>)
                    n217 = local read "DI Task"() -> (w76:refnum<k21>)
                    n218 = call "LookForPreInstHold.vi"("Home reward"="Home reward", "Home reward?"="Home reward?", "DI Task"=w76, "Touch lines"=w84, "Touching home\nlast time?"=w83, "Just initialized\nhold loop?"=w81, "Composite time"=w85, "DO Task"=w77) -> ("Touching home\nthis time?"=w82:bool, "Just initialized\nhold loop out?"=w80:bool, "Next stage in trial"=w86:T8)  [unwired: 1 in]
                    n219 = local write "Touching target\nlast time?"(w82) -> ()
                    n220 = local write "Just initialized\nhold loop?"(w80) -> ()
                  }
                  frame True {
                    n221 = while {
                      stop <- w88 continue-if-true
                      n222 = local read "pause"() -> (w88:bool)
                      n223 = Wait (ms)(milliseconds to wait=u32 100) -> ()  [unwired: 1 out]
                    }
                  }
                }
                n224 = local read "Exp reset"() -> (w73:bool)
              }
              frame "Instruction init" {
                n225 = stacked-sequence {
                  tunnel: w90 -> [_ _ w100 w101 _ _ _]
                  frame #0 {
                    n226 = local read "DO Task"() -> (w93:refnum<k21>)
                    n227 = call "WriteDigioBits2_DAQmx.vi"("Bits to write"=Bits_to_Write."In trial on", "DO Task"=w93) -> ()  [unwired: 9 in, 1 out]
                  }
                  frame #1 {
                    n228 = local read "Record flag"() -> (w95:bool)
                    n229 = case shown="True" w95 {
                      frame False {
                      }
                      frame True {
                        n230 = local read "Exp trials"() -> (w99:i32)
                        n231 = local read "DO Task"() -> (w97:refnum<k21>)
                        n232 = Increment(x=w99) -> (x+1=w96:i32)
                        n233 = call "WriteDigioBits2_DAQmx.vi"("Bits to write"=Bits_to_Write."Trial number", "Number"=w96, "DO Task"=w97) -> ()  [unwired: 8 in, 1 out]
                      }
                    }
                  }
                  frame #2 {
                    "Target" <- w100
                  }
                  frame #3 {
                    n234 = local read "DO Task"() -> (w102:refnum<k21>)
                    n235 = call "WriteDigioBits2_DAQmx.vi"("Bits to write"=Bits_to_Write."Target number", "Number"=w101, "DO Task"=w102) -> ()  [unwired: 8 in, 1 out]
                  }
                  frame #4 {
                    n236 = case shown="1" "Trial type" {
                      tunnel: [Bits_to_Write."Trial type preQ off" ("Bits to write") Bits_to_Write."Trial type preQ on" ("Bits to write")] -> w104
                      frame 0, Default {
                        # "Trial type = all flash"
                      }
                      frame 1 {
                        # "Trial type = precue"
                      }
                    }
                    n237 = local read "DO Task"() -> (w105:refnum<k21>)
                    n238 = call "WriteDigioBits2_DAQmx.vi"("Bits to write"=w104, "DO Task"=w105) -> ()  [unwired: 9 in, 1 out]
                  }
                  frame #5 {
                    n239 = call "CalculateFixedPlusRandom2.vi"("Component times"="LED I duration") -> ("Composite time"=w109:dbl)  [unwired: 1 in, 1 out]
                    "Instruct duration" <- w109
                    n240 = Greater Than 0?(x=w109) -> (x > 0?=w110:bool)
                    n241 = case shown="True" w110 {
                      frame False {
                      }
                      frame True {
                        w117 = TRUE  # Initialize?
                        n242 = local read "Pre-cue brightness"() -> (w115:i16)
                        n243 = local read "All Flash?"() -> (w114:bool)
                        n244 = local read "DO Task"() -> (w113:refnum<k21>)
                        n245 = local read "DI Task"() -> (w112:refnum<k21>)
                        n246 = local read "Target"() -> (w116:i16)
                        n247 = call "Instruction.vi"("Initialize?"=w117, "DI Task"=w112, "All Flash?"=w114, "brightness"=w115, "Target"=w116, "DO Task"=w113) -> ()  [unwired: 4 in, 2 out]
                      }
                    }
                  }
                  frame #6 {
                    n248 = local read "Bumps"() -> (w118:bool)
                    n249 = local write "Start bump timer?"(w118) -> ()
                  }
                }
              }
              frame "Instruction" {
                w128 = FALSE  # Initialize?
                n250 = local read "Instruct duration"() -> (w124:dbl)
                n251 = local read "Touch lines"() -> (w129:T7)
                n252 = local read "DO Task"() -> (w120:refnum<k21>)
                n253 = local read "DI Task"() -> (w119:refnum<k21>)
                n254 = local read "Target"() -> (w126:i16)
                n255 = call "Instruction.vi"("Initialize?"=w128, "DI Task"=w119, "All Flash?"="All Flash?", "Touch lines"=w129, "Instruction duration"=w124, "brightness"="Pre-cue brightness", "Target"=w126, "DO Task"=w120) -> ("Last trial successful?"=w127:bool, "Go to stage"=w123:T8)  [unwired: 2 in]
                n256 = local write "Last trial successful?"(w127) -> ()
              }
              frame "Post-instruction hold init" {
                w135 = TRUE  # Initialize?
                n257 = local read "DI Task"() -> (w136:refnum<k21>)
                n258 = call "LookForPostInstHold.vi"("Initialize?"=w135, "Post-I \nbounce-off"="Post-I \nbounce-off", "Post-I hold"="Post-I hold", "DI Task"=w136) -> ("Last trial successful?"=w134:bool, "Go to stage"=w131:T8)  [unwired: 6 in]
                n259 = local write "Last trial successful?"(w134) -> ()
              }
              frame "Post-instruction hold" {
                w140 = FALSE  # Initialize?
                # "This is to clear our Catch Boolean during\nthe reward cycle. We put it here so it was\non long enough for us to catch."
                n260 = local read "Touch lines"() -> (w142:T7)
                n261 = local read "DI Task"() -> (w141:refnum<k21>)
                n262 = local write "Catch Trial?"(FALSE) -> ()
                n263 = call "LookForPostInstHold.vi"("Initialize?"=w140, "Touch lines"=w142, "DI Task"=w141) -> ("Last trial successful?"=w139:bool, "Go to stage"=w143:T8)  [unwired: 7 in]
                n264 = local write "Last trial successful?"(w139) -> ()
              }
              frame "Target capture init" {
                w153 = TRUE  # Initialize?
                n265 = local read "DO Task"() -> (w145:refnum<k21>)
                n266 = local read "DI Task"() -> (w144:refnum<k21>)
                n267 = local read "Target"() -> (w151:i16)
                n268 = call "TargetCapture.vi"("DO Task"=w145, "DI Task"=w144, "Response time"="Capture timeout", "Tone duration"="Tone duration", "LED C duration"="LED C duration", "Target"=w151, "Cue brightness"="Cue brightness", "Initialize?"=w153) -> ("Last trial successful?"=w149:bool)  [unwired: 6 in, 1 out]
                n269 = local write "Last trial successful?"(w149) -> ()
              }
              frame "Target capture" {
                w159 = FALSE  # Initialize?
                n270 = local read "Touch lines"() -> (w160:T7)
                n271 = local read "DO Task"() -> (w156:refnum<k21>)
                n272 = local read "DI Task"() -> (w155:refnum<k21>)
                n273 = local read "Target"() -> (w162:i16)
                n274 = call "TargetCapture.vi"("DO Task"=w156, "Touch lines"=w160, "DI Task"=w155, "Home+target OK?"="Home+target OK?", "Target"=w162, "Initialize?"=w159) -> ("Go to stage"=w163:T8, "Last trial successful?"=w161:bool)  [unwired: 8 in]
                n275 = local write "Last trial successful?"(w161) -> ()
              }
              frame "Target hold init" {
                w169 = TRUE  # Initialize?
                n276 = local read "DO Task"() -> (w165:refnum<k21>)
                n277 = local read "DI Task"() -> (w164:refnum<k21>)
                n278 = local read "Target"() -> (w167:i16)
                n279 = call "TargetHold.vi"("DO Task"=w165, "DI Task"=w164, "target hold"="Hold duration", "target\nbounce-off"="Allowed\nbounce-off", "Target"=w167, "Post-capture brightness"="Post-capture brightness", "Initialize?"=w169) -> ()  [unwired: 7 in, 2 out]
              }
              frame "Target hold" {
                w176 = FALSE  # Initialize?
                n280 = local read "Home+target OK?"() -> (w174:bool)
                n281 = local read "Touch lines"() -> (w179:T7)
                n282 = local read "DO Task"() -> (w180:refnum<k21>)
                n283 = local read "DI Task"() -> (w173:refnum<k21>)
                n284 = local read "Target"() -> (w178:i16)
                n285 = call "TargetHold.vi"("DO Task"=w180, "Touch lines"=w179, "DI Task"=w173, "Home+target OK?"=w174, "Target"=w178, "Initialize?"=w176) -> ("Go to stage"=w181:T8, "Last trial successful?"=w177:bool)  [unwired: 8 in]
                n286 = local write "Last trial successful?"(w177) -> ()
              }
              frame "Reward stage" {
                n287 = stacked-sequence {
                  frame #0 {
                    # "This will be a bit written in the \ndata file so we're not worried about \nit reseting."
                    n288 = Random Number (0-1)() -> (number: 0 to 1=w188:dbl)
                    n289 = Multiply(x=w188, y=100.0) -> (x*y=w187:dbl)
                    n290 = To Unsigned Long Integer(number=w187) -> (unsigned 32bit integer=w185:u32)
                    n291 = Less Or Equal?(x=w185, y="Catch probability") -> (x <= y?=w190:bool)
                    n292 = case shown="False" w190 {
                      selector: w190 -> [w194 w196]
                      tunnel: ["Reward duration" cluster{"Fix":dbl, "Rnd":dbl} {"Fix"=0.0, "Rnd"=0.0} ("Reward duration")] -> w192
                      tunnel: [w194 w196] -> w184
                      frame False {
                        # "Sending False bit for \ncatch trial"
                        # "Normal reward duration"
                      }
                      frame True {
                        # "Sending True bit for \ncatch trial"
                        # "This is the catch trial. \nSo we don't want to deliver \na reward"
                      }
                    }
                    "Catch Trial?" <- w184
                    n293 = call "CalculateFixedPlusRandom2.vi"("Component times"=w192) -> ("time in ms"=w193:dbl)  [unwired: 1 in, 1 out]
                    n294 = local read "DO Task"() -> (w191:refnum<k21>)
                    n295 = call "Reward Pulse.vi"("Pulse duration (ms)"=w193, "DO Task"=w191) -> ()  [unwired: 8 in]
                  }
                  frame #1 {
                    n296 = case shown="True" "Use Arm Freeze Counter" {
                      tunnel: _ -> [_ _]
                      frame False {
                      }
                      frame True {
                        n297 = while {
                          stop <- w203 stop-if-true
                          # "This case structure is to control a timer on the \nfront panel that counts to 5 seconds before moving\nthe monkey's hand back to the start key."
                          n298 = Tick Count (ms)() -> (millisecond timer value=w199:u32)
                          n299 = Multiply(x=w199, y=1000) -> (x*y=→"Arm Freeze Counter":u32)
                          n300 = Equal?(x=5000.0 ("Time Target (s)"), y=w199) -> (x = y?=w203:bool)
                        }
                      }
                    }
                  }
                }
              }
              frame "Intertrial" {
                n301 = local read "Last trial successful?"() -> (w221:bool)
                n302 = local read "Bumps"() -> (w205:bool)
                n303 = local read "target set size"() -> (w209:i32)
                n304 = local read "# target sets"() -> (w210:u16)
                n305 = call "CalculateFixedPlusRandom2.vi"("Component times"="Intertrial interval") -> ("Composite time"=w222:dbl)  [unwired: 1 in, 1 out]
                n306 = local write "Override bumps"(w205) -> ()
                n307 = local write "Recenter motor"(w205) -> ()
                n308 = while {
                  shift-right: [enum16{"Start counting", "Read count", "Reset"}."Read count" ("Enum")] -> _
                  shift-left: enum16{"Start counting", "Read count", "Reset"}."Start counting" ("Enum") -> [w240]
                  tunnel: [w235] -> _
                  tunnel: w222 -> [w234]
                  stop <- w236 stop-if-true
                  n309 = call "non-Reentrant Controllable Timer.vi"("Enum"=w240) -> ("Time out"=w238:dbl)  [unwired: 1 in]
                  n310 = local read "stop"() -> (w237:bool)
                  n311 = Greater Or Equal?(x=w238, y=w234) -> (x >= y?=w235:bool)
                  n312 = Or(x=w235, y=w237) -> (x .or. y?=w236:bool)
                }
                n313 = Multiply(x=w210, y=w209) -> (x*y=w208:i32)
                n314 = call "TrackStats2.vi"("Last trial successful?"=w221, "Trial bin size"=w208, "Persistent\n Mode?"="Persistent\n Mode?", "Command"=enum16{"Reset", "Increment"}."Increment") -> ("Total incorrect"=→"Total incorrect":i32, "Total correct"=→"Total correct":i32, "# total trials"=→"Total trials":i32, "Total % correct"=w213:dbl, "Segment trials"=→"Block trials":i32, "Experiment trials"=→"Exp trials":i32, "Experiment correct"=→"Exp correct":i32, "Experiment %"=→"Exp %":dbl, "Segment Percentage"=w214:dbl)  [unwired: 3 in]
                "Block %" <- w214
                "Total %" <- w213
                n315 = Bundle("Segment Percentage"=w214, "Total % correct"=w213) -> (→"Waveform Chart":T6)  [unwired: 1 in]
                n316 = stacked-sequence {
                  frame #0 {
                    n317 = local read "Last trial successful?"() -> (w227:bool)
                    n318 = case shown="True" w227 {
                      frame False {
                        n319 = local read "DO Task"() -> (w228:refnum<k21>)
                        n320 = call "Signal Error.vi"("DO Task"=w228, "Error bong?"="Error\nbong?") -> ()  [unwired: 3 in]
                      }
                      frame True {
                      }
                    }
                  }
                  frame #1 {
                    n321 = local read "DO Task"() -> (w230:refnum<k21>)
                    n322 = call "WriteDigioBits2_DAQmx.vi"("Bits to write"=Bits_to_Write."In trial off", "DO Task"=w230) -> ()  [unwired: 9 in, 1 out]
                  }
                  frame #2 {
                  }
                }
                n323 = local read "Persistent\n Mode?"() -> (w211:bool)
                n324 = case shown="False" w211 {
                  tunnel: [w232 w233] -> w225
                  frame False {
                    w232 = TRUE  # End of trial
                  }
                  frame True {
                    n325 = local read "Last trial successful?"() -> (w233:bool)
                  }
                }
              }
            }
            n326 = Wait (ms)(milliseconds to wait=u32 1) -> ()  [unwired: 1 out]
            n327 = Compound Arithmetic op=OR(w63, "stop") -> (w61:bool)
            "Current stage" <- w65
          }
          n328 = local read "Exp reset"() -> (w51:bool)
          n329 = Compound Arithmetic op=OR(w53, w52, w51) -> (w50:bool)
        }
        n330 = Or(x=w48, y=w47) -> (x .or. y?=w46:bool)
      }
    }
    frame #3 {
      # "Turn LED's, \nbuzzer,\npump off\njust to be\nsure"
      n331 = local read "DO Task"() -> (w413:refnum<k21>)
      n332 = local read "DO Task"() -> (w411:refnum<k21>)
      n333 = local read "DO Task"() -> (w415:refnum<k21>)
      n334 = local read "DO Task"() -> (w416:refnum<k21>)
      n335 = local read "DO Task"() -> (w418:refnum<k21>)
      n336 = local read "DO Task"() -> (w420:refnum<k21>)
      n337 = local write "Record flag"(FALSE ("Record flag")) -> ()
      n338 = call "WriteDigioBits2_DAQmx.vi"("Bits to write"=Bits_to_Write."In trial off", "DO Task"=w413) -> ()  [unwired: 9 in, 1 out]
      n339 = call "WriteDigioBits2_DAQmx.vi"("Bits to write"=Bits_to_Write."All LEDs off", "DO Task"=w411) -> ()  [unwired: 9 in, 1 out]
      n340 = call "WriteDigioBits2_DAQmx.vi"("Bits to write"=Bits_to_Write."Buzzer off", "DO Task"=w415) -> ()  [unwired: 9 in, 1 out]
      n341 = call "WriteDigioBits2_DAQmx.vi"("Bits to write"=Bits_to_Write."Reward off", "DO Task"=w416) -> ()  [unwired: 9 in, 1 out]
      n342 = call "WriteDigioBits2_DAQmx.vi"("Bits to write"=Bits_to_Write."Error off", "DO Task"=w418) -> ()  [unwired: 9 in, 1 out]
      n343 = call "WriteDigioBits2_DAQmx.vi"("Bits to write"=Bits_to_Write."DBS off", "DO Task"=w420) -> ()  [unwired: 9 in, 1 out]
      n344 = local write "stop"(FALSE ("stop")) -> ()
    }
  }
